vi "Check Abnormal.vi"(9 "Known Found?":bool, 10 "Filenames":string[](array[string])) -> (1 "Ignore":bool, 2 "Filenames out":string[](array[string]))   [LabVIEW 2023]
uses:
  <vilib>/Analysis/NI_AALBase.lvlib
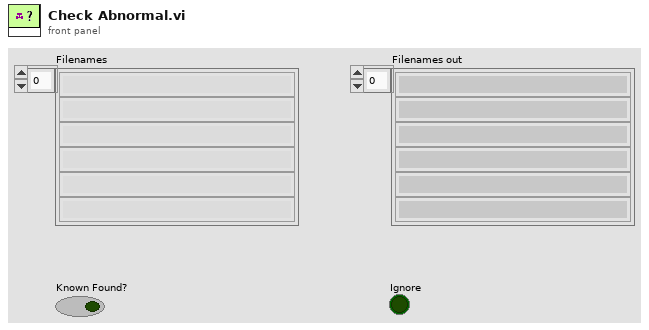
[diagram p1: front panel]
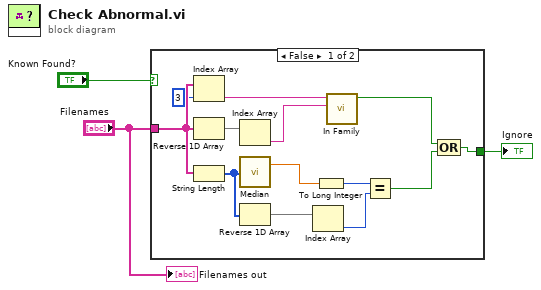
[diagram p0: block diagram]
diagram:
  n1 = case shown="False" "Known Found?" {
    tunnel: "Filenames" -> [w9 _]
    tunnel: [w10 _] -> w2
    frame False {
      n2 = Index Array(array=w9, index=3) -> (element=w7:string)
      n3 = Reverse 1D Array(array=w9) -> (reversed array=w12:string[])
      n4 = String Length(string=w9) -> (length=w16:i32[])
      n5 = Index Array(array=w12) -> (element=w6:string)  [unwired: 1 in]
      n6 = call <vilib>:"Median.vi"("X"=w16) -> ("median"=w11:dbl)  [unwired: 1 out]
      n7 = Reverse 1D Array(array=w16) -> (reversed array=w14:i32[])
      n8 = Index Array(array=w14) -> (element=w13:i32)  [unwired: 1 in]
      n9 = To Long Integer(number=w11) -> (32bit integer=w15:i32)
      n10 = call "In Family.vi"("String 2"=w6, "String 1"=w7) -> ("Family?"=w5:bool)  [unwired: 9 in]
      n11 = Equal?(x=w15, y=w13) -> (x = y?=w4:bool)
      n12 = Compound Arithmetic op=OR(w5, w4) -> (w10:bool)
    }
    frame True {
    }
  }
  "Ignore" <- w2
  "Filenames out" <- "Filenames"
